vi "Configure.vi"(8 "error in":errorcluster, 11 "Control Load CFG in":refnum<class "EL Control Load CFG.lvclass">) -> (0 "error out":errorcluster, 3 "Control Load CFG out":refnum<class "EL Control Load CFG.lvclass">)   [LabVIEW 2023, in "EL Control Load CFG.lvclass"]
uses:
  EL Control Load CFG.lvclass
  D:/git/HAL/HAL/Configurations/CFG JSON/CFG JSON.lvclass
  EL Control Load CFG.lvclass/EL Control Load CFG.ctl
  <vilib>/Utility/error.llb/Error Cluster From Error Code.vi
  <vilib>/ErrorRing/Error Ring.xnode
  <userlib>/_OpenG.lib/time/time.llb/openg_time.lvlib
  Configurations/CFG JSON/CFG JSON.lvclass
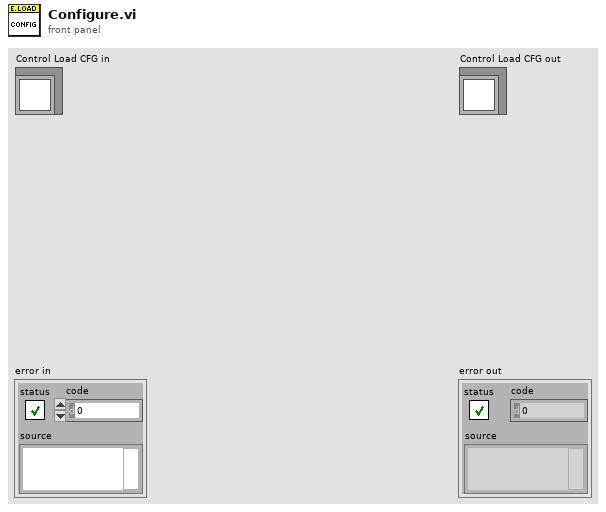
[diagram p1: front panel]
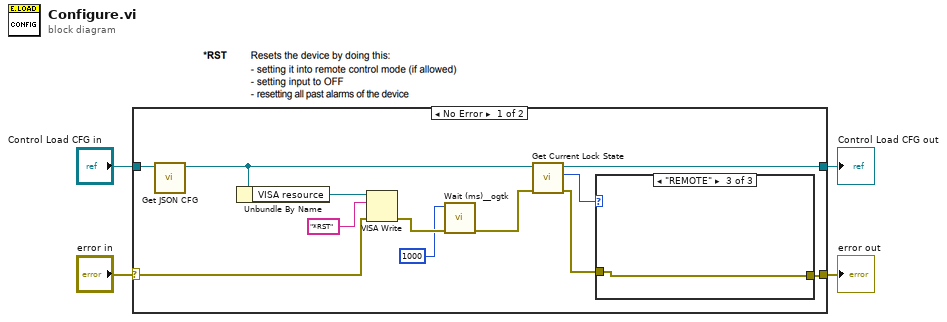
[diagram p0: block diagram]
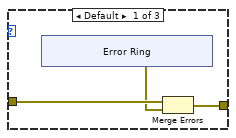
[diagram p2: hidden frame]
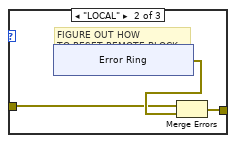
[diagram p3: hidden frame]
diagram:
  n1 = case shown="No Error" "error in" {
    selector: "error in" -> [w11 w35]
    tunnel: [w6 w35] -> w3
    tunnel: [w8 w34] -> w1
    tunnel: "Control Load CFG in" -> [w16 w34]
    frame No Error {
      n2 = call "Get JSON CFG.vi"("CFG JSON in"=w16) -> ("CFG JSON out"=w9:refnum<class "EL Control Load CFG.lvclass">)  [unwired: 9 in, 1 out]
      n3 = Unbundle By Name(w9) -> ("VISA resource"=w15:refnum<visa-resource-name>)
      n4 = VISA Write(VISA resource name=w15, write buffer="*RST", error in (no error)=w11) -> (error out=w13:errorcluster)  [unwired: 2 out]
      n5 = call <userlib>:"Wait (ms)__ogtk.vi"("error in (no error)"=w13, "milliseconds to wait"=u32 1000) -> ("error out"=w10:errorcluster)  [unwired: 8 in, 1 out]
      n6 = call "Get Current Lock State.vi"("error in"=w10, "EL Control Load CFG in"=w9) -> ("error out"=w5:errorcluster, "Lock State"=w7:enum16{"NONE", "LOCAL", "REMOTE"}, "EL Control Load CFG out"=w8:refnum<class "EL Control Load CFG.lvclass">)  [unwired: 7 in]
      n7 = case shown="\"REMOTE\"" w7 {
        tunnel: [w19 w27 w33] -> w6
        tunnel: w5 -> [w18 w25 w33]
        frame Default {
          n8 = xnode "Error Ring"() -> ("error out"=w17:errorcluster)
          n9 = Merge Errors(w18, w17) -> (w19:errorcluster)
        }
        frame "LOCAL" {
          # "FIGURE OUT HOW\nTO RESET REMOTE BLOCK"
          n10 = xnode "Error Ring"() -> ("error out"=w26:errorcluster)
          n11 = Merge Errors(w25, w26) -> (w27:errorcluster)
        }
        frame "REMOTE" {
        }
      }
    }
    frame Error {
    }
  }
  "error out" <- w3
  "Control Load CFG out" <- w1
